vi "GaussianRandomProjection.vi"(8 "error in":errorcluster caption="entrée d'erreur", 11 "GaussianRandomProjection":T1={"n_components"="auto", "eps"=0.1, "random_state"=-1} {"random_state" min=-1; "eps" min=0.0}) -> (0 "error out":errorcluster caption="sortie d'erreur", 3 "GaussianRandomProjection.lvclass":refnum<class "GaussianRandomProjection.lvclass">)   [LabVIEW 2020]
doc: "Reduce dimensionality through Gaussian random projection\n\nThe components of the random matrix are drawn from N(0, 1 / n_components).\n\nParameters : \n\n- n_components : int or ‘auto’, optional (default = ‘auto’)\nDimensionality of the target projection space.\n\nn_components can be automatically adjusted according to the number of samples in the dataset and the bound given by the Johnson-Lindenstrauss lemma. In that case the quality of the embedding is controlled by the eps parameter.\n\nIt should be noted that Johnson-Lindenstrauss lemma can yield very conservative estimated of the required number of components as it makes no assumption on the structure of the dataset.\n\n- eps : strictly positive float, optional=None=-1 (default=0.1)\nParameter to control the quality of the embedding according to the Johnson-Lindenstrauss lemma when n_components is set to ‘auto’.\n\nSmaller values lead to better embedding and higher number of dimensions (n_components) in the target projection space.\n\n- random_state : int, RandomState instance or None, optional (default=None=-1)\nControls the pseudo random number generator used to generate the projection matrix at fit time. Pass an int for reproducible output across multiple function calls. \n\n\nMethods :\n\n- Fit : Generate a sparse random projection matrix\n\nParameters : X : numpy array or scipy.sparse of shape [n_samples, n_features]\n Training set: only the shape is used to find optimal random matrix dimensions based on the theory referenced in the afore mentioned papers.\n y : Ignored\n\n\n- Fit Transform : Fit to data, then transform it. Fits transformer to X and y with optional parameters fit_params and returns a transformed version of X.\n\nParameters : X : {array-like, sparse matrix, dataframe} of shape (n_samples, n_features)\n y : ndarray of shape (n_samples,), default=None\n Target values.\n\nReturns : X_newn : darray array of shape (n_samples, n_features_new)\n Transformed array.\n\n\n- Transform : Project the data by using matrix product with the random matrix\n\nParameters : X : numpy array or scipy.sparse of shape [n_samples, n_features]\n The input data to project into a smaller dimensional space.\n\nReturns : X_new : numpy array or scipy sparse of shape [n_samples, n_components]\n Projected array."
uses:
  GaussianRandomProjection.lvclass
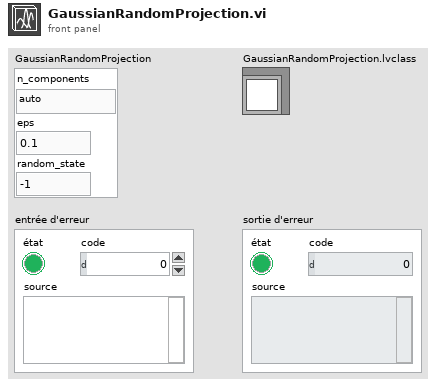
[diagram p1: front panel]
types:
  T1 = cluster{"n_components":string, "eps":dbl, "random_state":i32}
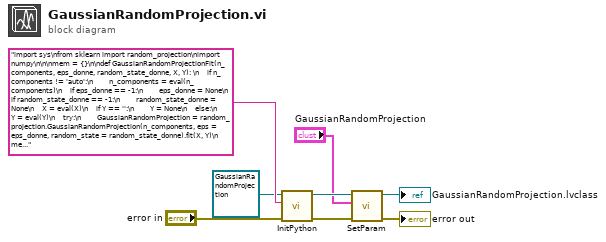
[diagram p0: block diagram]
diagram:
  n1 = call-dynamic "InitPython.vi"("error in (no error)"="error in", "Python Instruction"="import sys\nfrom sklearn import random_projection\nimport numpy\n\n\nmem = {}\n\ndef GaussianRandomProjectionFit(n_components, eps_donne, random_state_donne, X, Y): \n    if n_components != 'auto':\n        n_components = eval(n_components)\n    if eps_donne == -1:\n        eps_donne = None\n    if random_state_donne == -1:\n        random_state_donne = None\n    X = eval(X)\n    if Y == '':\n        Y = None\n    else:\n        Y = eval(Y)\n    try:\n        GaussianRandomProjection = random_projection.GaussianRandomProjection(n_components, eps = eps_donne, random_state = random_state_donne).fit(X, Y)\n        mem['FitGaussianRandomProjection'] = GaussianRandomProjection\n        return str('OK')\n    except:\n        erreur = sys.exc_info()\n        typerr = u\"%s\" % (erreur[0])\n        typerr = typerr[typerr.find(\"'\")+1:typerr.rfind(\"'\")]\n        msgerr = u\"%s\" % (erreur[1])\n        message = str('/!\\\\ {0} : {1}'. format(typerr,msgerr))\n        return message \n\ndef GaussianRandomProjectionFitTransform(n_components, eps_donne, random_state_donne, X, Y):\n    if n_components != 'auto':\n        n_components = eval(n_components)\n    if eps_donne == -1:\n        eps_donne = None\n    if random_state_donne == -1:\n        random_state_donne = None\n    X = eval(X)\n    if Y == '':\n        Y = None\n    else:\n        Y = eval(Y)\n    try:\n        GaussianRandomProjection = random_projection.GaussianRandomProjection(n_components, eps = eps_donne, random_state = random_state_donne).fit_transform(X, Y)\n        dtype = type(GaussianRandomProjection)\n        if dtype == numpy.ndarray:\n            GaussianRandomProjection = GaussianRandomProjection.tolist()\n            return str(GaussianRandomProjection)\n        else:\n            Mat = GaussianRandomProjection.tocoo()\n            return str(list(zip(Mat.row, Mat.col, Mat.data)))\n    except:\n        erreur = sys.exc_info()\n        typerr = u\"%s\" % (erreur[0])\n        typerr = typerr[typerr.find(\"'\")+1:typerr.rfind(\"'\")]\n        msgerr = u\"%s\" % (erreur[1])\n        message = str('/!\\\\ {0} : {1}'. format(typerr,msgerr))\n        return message \n    \n\ndef GaussianRandomProjectionTransform(n_components, eps_donne, random_state_donne, X, Y):\n    if n_components != 'auto':\n        n_components = eval(n_components)\n    if eps_donne == -1:\n        eps_donne = None\n    if random_state_donne == -1:\n        random_state_donne = None\n    X = eval(X)\n    if Y == '':\n        Y = None\n    else:\n        Y = eval(Y)\n    try:\n        GaussianRandomProjection = mem['FitGaussianRandomProjection'].transform(X, Y)\n        dtype = type(GaussianRandomProjection)\n        if dtype == numpy.ndarray:\n            GaussianRandomProjection = GaussianRandomProjection.tolist()\n            return str(GaussianRandomProjection)\n        else:\n            Mat = GaussianRandomProjection.tocoo()\n            return str(list(zip(Mat.row, Mat.col, Mat.data)))\n    except:\n        erreur = sys.exc_info()\n        typerr = u\"%s\" % (erreur[0])\n        typerr = typerr[typerr.find(\"'\")+1:typerr.rfind(\"'\")]\n        msgerr = u\"%s\" % (erreur[1])\n        message = str('/!\\\\ {0} : {1}'. format(typerr,msgerr))\n        return message", "Scikit-learn en entrée"=refnum<class "GaussianRandomProjection.lvclass"> refnum ("GaussianRandomProjection.lvclass")) -> ("error out"=w4:errorcluster, "Scikit-learn en sortie"=w5:refnum<class "GaussianRandomProjection.lvclass">)  [unwired: 7 in]
  n2 = call-dynamic "SetParam.vi"("error in (no error)"=w4, "GaussianRandomProjection"="GaussianRandomProjection", "GaussianRandomProjection.lvclass"=w5) -> ("error out"=→"error out":errorcluster, "GaussianRandomProjection.lvclass"=→"GaussianRandomProjection.lvclass":refnum<class "GaussianRandomProjection.lvclass">)  [unwired: 7 in]
